vi "String ist eine gueltige Zahl.vi"(11 "String":string) -> (3 "Zahl":bool)   [LabVIEW 2020, in "Linearisierung v2.lvlib"]
uses:
  Linearisierung v2.lvlib
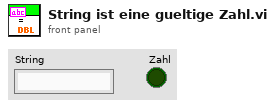
[diagram p1: front panel]
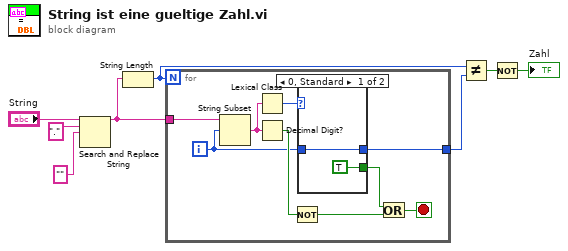
[diagram p0: block diagram]
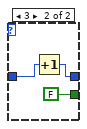
[diagram p2: hidden frame]
diagram:
  n1 = Search and Replace String(input string="String", search string="." ("Ersetzungs-String (\"\")"), replace string="" ("Ersetzungs-String (\"\")")) -> (result string=w5:string)  [unwired: 5 in, 3 out]
  n2 = String Length(string=w5) -> (length=w7:i32)
  n3 = for {
    N: w7 -> [_]
    tunnel: w5 -> [w17]
    tunnel: [w9] -> w8
    i -> [w10]
    stop <- w11 stop-if-true
    n4 = String Subset(string=w17, offset (0)=w10) -> (substring=w15:string)  [unwired: 1 in]
    n5 = Lexical Class(1:w15) -> (0:w14:i16)
    n6 = Decimal Digit?(1:w15) -> (0:w16:bool)
    n7 = Not(x=w16) -> (.not. x?=w13:bool)
    n8 = case shown="0, Standard" w14 {
      tunnel: [TRUE FALSE] -> w12
      tunnel: w10 -> [w18 w21]
      tunnel: [w18 w20] -> w9
      frame 0, Default {
      }
      frame 3 {
        n9 = Increment(x=w21) -> (x+1=w20:i32)
      }
    }
    n10 = Or(x=w12, y=w13) -> (x .or. y?=w11:bool)
  }
  n11 = Not Equal?(x=w7, y=w8) -> (x != y?=w6:bool)
  n12 = Not(x=w6) -> (.not. x?=→"Zahl":bool)
